vi "Utility MODBUS RTU Send Message.vi"(0 "VISA resource name":refnum<visa-resource-name>, 1 "Unit Address (1)":u8=1, 5 "Message (empty array)":u8[](array[numeric]), 11 "error in (no error)":errorcluster, 12 "Command (0)":u8) -> (4 "VISA resource name out":refnum<visa-resource-name>, 6 "Length Of Sent MSG":u8, 15 "error out":errorcluster)   [LabVIEW 2010, in "Eurotherm 32xx Series.lvlib"]
doc: "This VI sends the MODBUS message."
uses:
  <instrlib>/Eurotherm 32xx Series/Eurotherm 32xx Series.lvlib
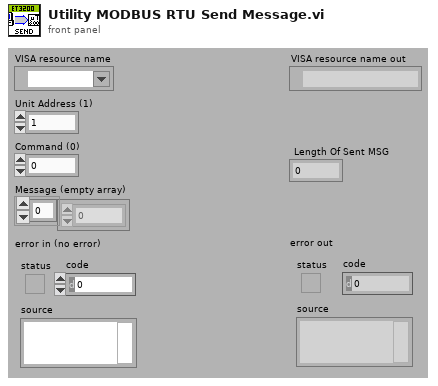
[diagram p1: front panel]
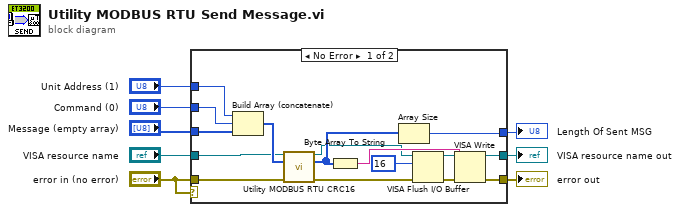
[diagram p0: block diagram]
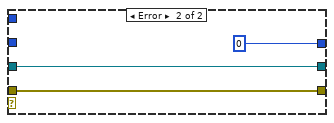
[diagram p2: hidden frame]
diagram:
  n1 = case shown="No Error" "error in (no error)" {
    tunnel: "error in (no error)" -> [w24 w26]
    tunnel: [w14 w26] -> w8
    tunnel: [w15 w27] -> w7
    tunnel: "Command (0)" -> [w23 _]
    tunnel: "Unit Address (1)" -> [w22 _]
    tunnel: "VISA resource name" -> [w20 w27]
    tunnel: [w19 0] -> w3
    tunnel: "Message (empty array)" -> [w17 _]
    frame No Error {
      n2 = Build Array (concatenate)(w22, w23, w17) -> (w21:u8[])
      n3 = call <instrlib>:"Utility MODBUS RTU CRC16.vi"("VISA resource name"=w20, "Message (empty array)"=w21, "error in (no error)"=w24) -> ("VISA resource name out"=w12:refnum<visa-resource-name>, "Message with CRC"=w18:u8[], "error out"=w11:errorcluster)  [unwired: 9 in, 1 out]
      n4 = Byte Array To String(unsigned byte array=w18) -> (string=w16:string)
      n5 = Array Size(array=w18) -> (size(s)=w19:i32)
      n6 = VISA Flush I/O Buffer(VISA resource name=w12, mask (16)=u16 16, error in (no error)=w11) -> (VISA resource name out=w13:refnum<visa-resource-name>, error out=w10:errorcluster)
      n7 = VISA Write(VISA resource name=w13, write buffer=w16, error in (no error)=w10) -> (VISA resource name out=w15:refnum<visa-resource-name>, error out=w14:errorcluster)  [unwired: 1 out]
    }
    frame Error {
    }
  }
  "error out" <- w8
  "VISA resource name out" <- w7
  "Length Of Sent MSG" <- w3
